vi "Get Port.vi"(8 "error in (no error)":errorcluster, 11 "Instrument.Example in":refnum<class "Instrument.Example.lvclass">) -> (0 "error out":errorcluster, 2 "port":u32, 3 "Instrument.Example out":refnum<class "Instrument.Example.lvclass">)   [LabVIEW 2016]
uses:
  Instrument.Example.lvclass
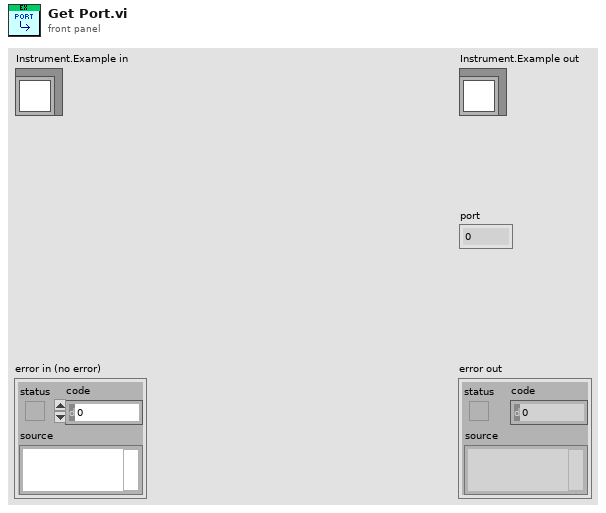
[diagram p1: front panel]
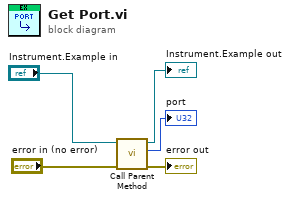
[diagram p0: block diagram]
diagram:
  n1 = call-parent "Call Parent Method"("error in (no error)"="error in (no error)", "Instrument in"="Instrument.Example in") -> ("error out"=→"error out":errorcluster, "port"=→"port":u32, "Instrument out"=→"Instrument.Example out":refnum<class "Instrument.Example.lvclass">)  [unwired: 7 in]
